vi "Main.vi"() -> ()   [LabVIEW 2014]
uses:
  <vilib>/Instr/_visa.llb/VISA Configure Serial Port (Instr).vi
panel:
  in  "Sim Delay":u32(slide)=100 scale=0.0..2000.0
  in  "조작모드":string(combo)="기본"
  out "Serial Loop":i32=157
  in  "Serial Settings":T1={"baud rate"=9600, "data bits"=8, "parity"=enum."None", "stop bits"=10, "flow control"=0} {"flow control" items=["None"=0, "XON/XOFF"=1, "RTS/CTS"=2, "DTR/DSR"=4]; "stop bits" items=["1.0"=10, "1.5"=15, "2.0"=20]; "data bits" min=5 max=8 step=1; "baud rate" items=["75"=75, "110"=110, "134"=134, "150"=150, "300"=300, "600"=600, "1200"=1200, "1800"=1800, "2400"=2400, "4800"=4800, "7200"=7200, "9600"=9600, "14400"=14400, "19200"=19200, "28800"=28800, "38400"=38400, "56000"=56000, "57600"=57600, "115200"=115200, "128000"=128000, "230400"=230400]}
  in  "VISA 2":refnum<visa-resource-name>="COM4"
  in  "VISA 1":refnum<visa-resource-name>="COM3"
  out "Running 2":bool=TRUE caption="Running"
  in  "재생 버튼":bool
  out "Running":bool=TRUE
  in  "Serial Delay":u32(slide)=1000 scale=0.0..2000.0
  out "C축":dbl(knob)=10.0 scale=0.0..10.0
  out "R축":dbl(knob) scale=0.0..10.0
  out "L축":dbl(knob) scale=0.0..10.0
  out "Wrtie":string
  out "Axis":string
  out "위치 좌표 값 그래프":dbl[][](graph)=[[127.0, 127.0, 127.0], [127.0, 127.0, 127.0], [127.0, 127.0, 127.0], [127.0, 127.0, 127.0], [127.0, 127.0, 127.0], [127.0, 127.0, 127.0], [127.0, 127.0, 127.0], [127.0, 127.0, 127.0], [127.0, 127.0, 127.0], [127.0, 127.0, 127.0], [127.0, 127.0, 127.0], [127.0, 127.0, 127.0], [127.0, 127.0, 127.0], [127.0, 127.0, 127.0], [127.0, 127.0, 127.0], [127.0, 127.0, 127.0], [127.0, 127.0, 127.0], [127.0, 127.0, 127.0], [127.0, 127.0, 127.0], [127.0, 127.0, 127.0], [127.0, 127.0, 127.0], [127.0, 127.0, 127.0], [127.0, 127.0, 127.0], [127.0, 127.0, 127.0], [127.0, 127.0, 127.0], [127.0, 127.0, 127.0], [127.0, 127.0, 127.0], [127.0, 127.0, 127.0], [127.0, 127.0, 127.0], [127.0, 127.0, 127.0], [127.0, 127.0, 127.0], [127.0, 127.0, 127.0], [127.0, 127.0, 127.0], [127.0, 127.0, 127.0], [127.0, 127.0, 127.0], [127.0, 127.0, 127.0], [127.0, 127.0, 127.0], [127.0, 127.0, 127.0], [127.0, 127.0, 127.0], [127.0, 127.0, 127.0], [127.0, 127.0, 127.0], [127.0, 127.0, 127.0], [127.0, 127.0, 127.0], [127.0, 127.0, 127.0], [127.0, 127.0, 127.0], [127.0, 127.0, 127.0], [127.0, 127.0, 127.0], [127.0, 127.0, 127.0], [127.0, 127.0, 127.0], [127.0, 127.0, 127.0], [127.0, 127.0, 127.0], [127.0, 127.0, 127.0], [127.0, 127.0, 127.0], [127.0, 127.0, 127.0], [127.0, 127.0, 127.0], [127.0, 127.0, 127.0], [127.0, 127.0, 127.0], [127.0, 127.0, 127.0], [127.0, 127.0, 127.0], [127.0, 127.0, 127.0], [127.0, 127.0, 127.0], [127.0, 127.0, 127.0], [127.0, 127.0, 127.0], [127.0, 127.0, 127.0], [127.0, 127.0, 127.0], [127.0, 127.0, 127.0], [127.0, 127.0, 127.0], [127.0, 127.0, 127.0], [127.0, 127.0, 127.0], [127.0, 127.0, 127.0], [127.0, 127.0, 127.0], [127.0, 127.0, 127.0], [127.0, 127.0, 127.0], [127.0, 127.0, 127.0], [127.0, 127.0, 127.0], [127.0, 127.0, 127.0], [127.0, 127.0, 127.0], [127.0, 127.0, 127.0], [127.0, 127.0, 127.0], [127.0, 127.0, 127.0], [127.0, 127.0, 127.0], [127.0, 127.0, 127.0], [127.0, 127.0, 127.0], [127.0, 127.0, 127.0], [127.0, 127.0, 127.0], [127.0, 127.0, 127.0], [127.0, 127.0, 127.0], [127.0, 127.0, 127.0], [127.0, 127.0, 127.0], [127.0, 127.0, 127.0], [127.0, 127.0, 127.0], [127.0, 127.0, 127.0], [127.0, 127.0, 127.0], [127.0, 127.0, 127.0], [127.0, 127.0, 127.0], [127.0, 127.0, 127.0], [127.0, 127.0, 127.0], [127.0, 127.0, 127.0], [127.0, 127.0, 127.0], [127.0, 127.0, 127.0], [127.0, 127.0, 127.0], [127.0, 127.0, 127.0], [127.0, 127.0, 127.0], [127.0, 127.0, 127.0], [127.0, 127.0, 127.0], [127.0, 127.0, 127.0], [127.0, 127.0, 127.0], [127.0, 127.0, 127.0], [127.0, 127.0, 127.0], [127.0, 127.0, 127.0], [127.0, 127.0, 127.0], [127.0, 127.0, 127.0], [127.0, 127.0, 127.0], [127.0, 127.0, 127.0], [127.0, 127.0, 127.0], [127.0, 127.0, 127.0], [127.0, 127.0, 127.0], [127.0, 127.0, 127.0], [127.0, 127.0, 127.0], [127.0, 127.0, 127.0], [127.0, 127.0, 127.0], [127.0, 127.0, 127.0], [127.0, 127.0, 127.0], [127.0, 127.0, 127.0], [127.0, 127.0, 127.0], [127.0, 127.0, 127.0], [127.0, 127.0, 127.0], [127.0, 127.0, 127.0], [127.0, 127.0, 127.0], [127.0, 127.0, 127.0], [127.0, 127.0, 127.0], [127.0, 127.0, 127.0], [127.0, 127.0, 127.0], [127.0, 127.0, 127.0], [127.0, 127.0, 127.0], [127.0, 127.0, 127.0], [127.0, 127.0, 127.0], [127.0, 127.0, 127.0], [127.0, 127.0, 127.0], [127.0, 127.0, 127.0], [127.0, 127.0, 127.0], [127.0, 127.0, 127.0], [127.0, 127.0, 127.0], [127.0, 127.0, 127.0], [127.0, 127.0, 127.0], [127.0, 127.0, 127.0], [127.0, 127.0, 127.0], [127.0, 127.0, 127.0], [127.0, 127.0, 127.0], [127.0, 127.0, 127.0], [127.0, 127.0, 127.0], [127.0, 127.0, 127.0], [127.0, 127.0, 127.0], [127.0, 127.0, 127.0], [127.0, 127.0, 127.0], [127.0, 127.0, 127.0], [127.0, 127.0, 127.0], [127.0, 127.0, 127.0]]
  in  "Error In":errorcluster
  in  "포트":u16=50
  in  "IP":string="127.0.0.1"
  in  "Running Game":string="DiRT 3"
  out "Sim Loop":i32=157
  in  "Simtools ON":bool
  in  "STOP":bool
  out "Error Out":errorcluster={"status"=TRUE, "code"=-1074360311, "source"="IMAQdx Open Camera.vi"}
  # "지도교수 : 손종원 교수님, 윤한재 교수님, 노일수 교수님  개발자 : 하기봉, 박재우"
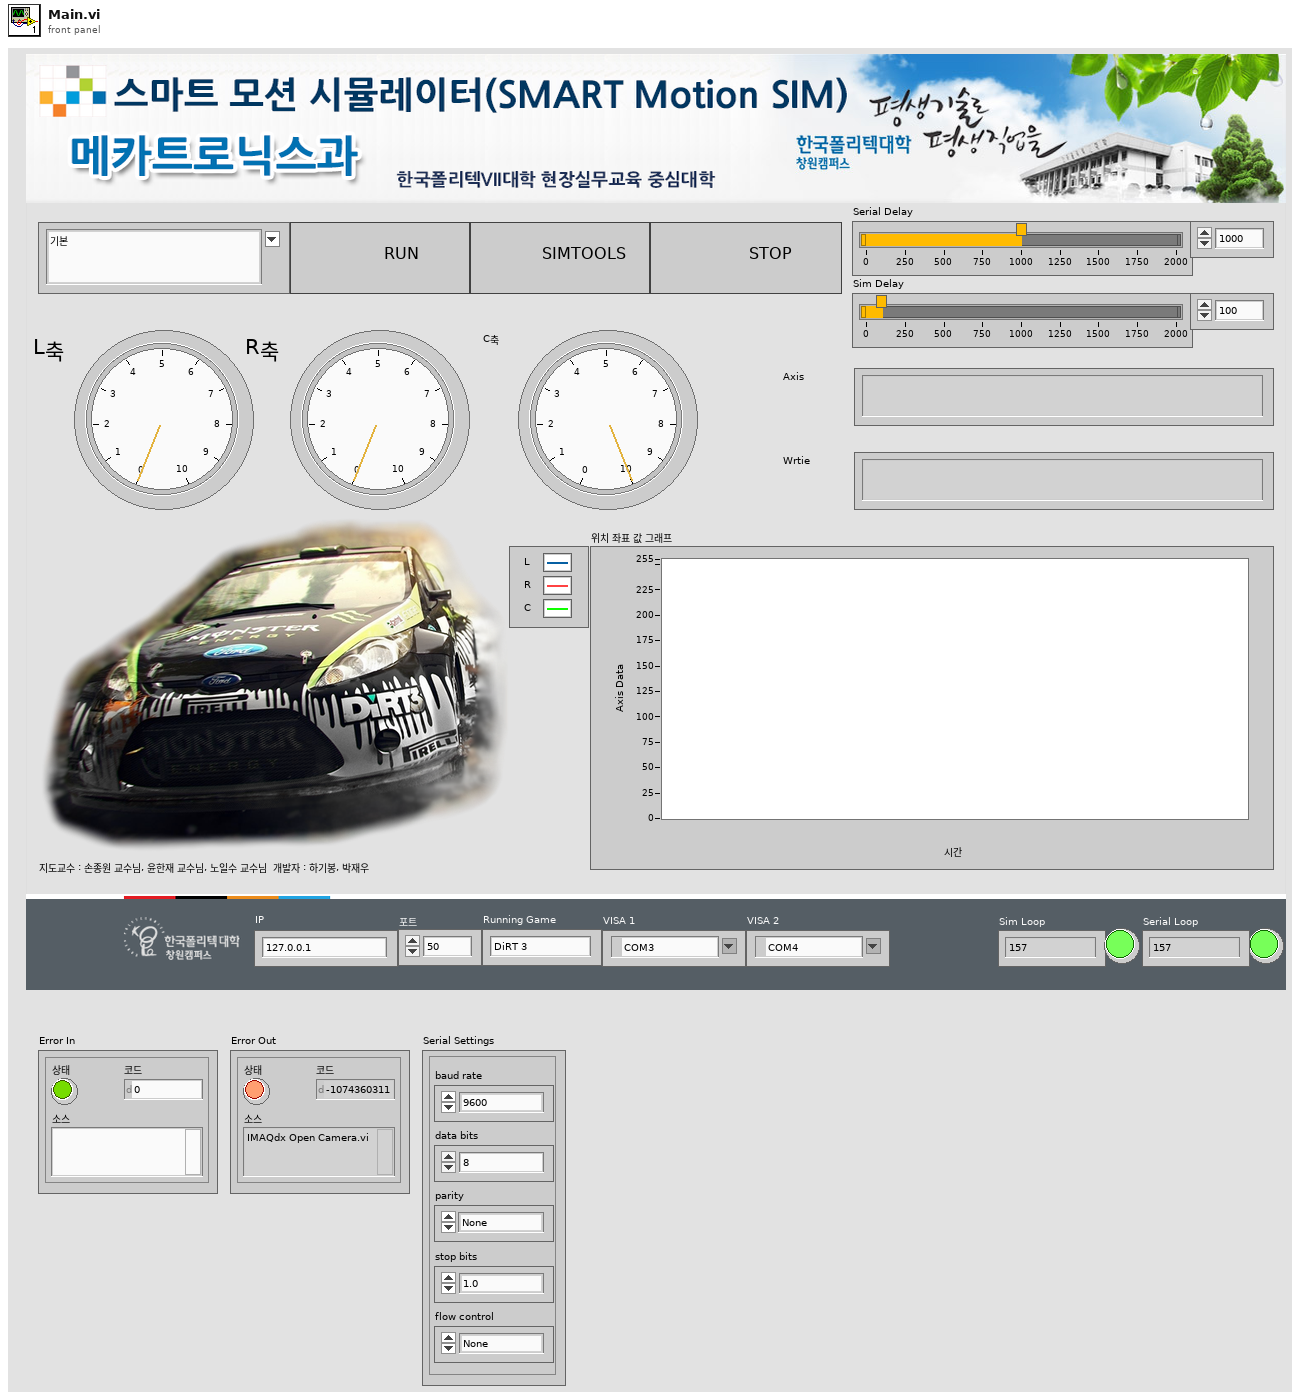
[diagram p1: front panel]
types:
  T1 = cluster{"baud rate":u32, "data bits":u16, "parity":enum16{"None", "Odd", "Even", "Mark", "Space"}, "stop bits":u16, "flow control":u16}
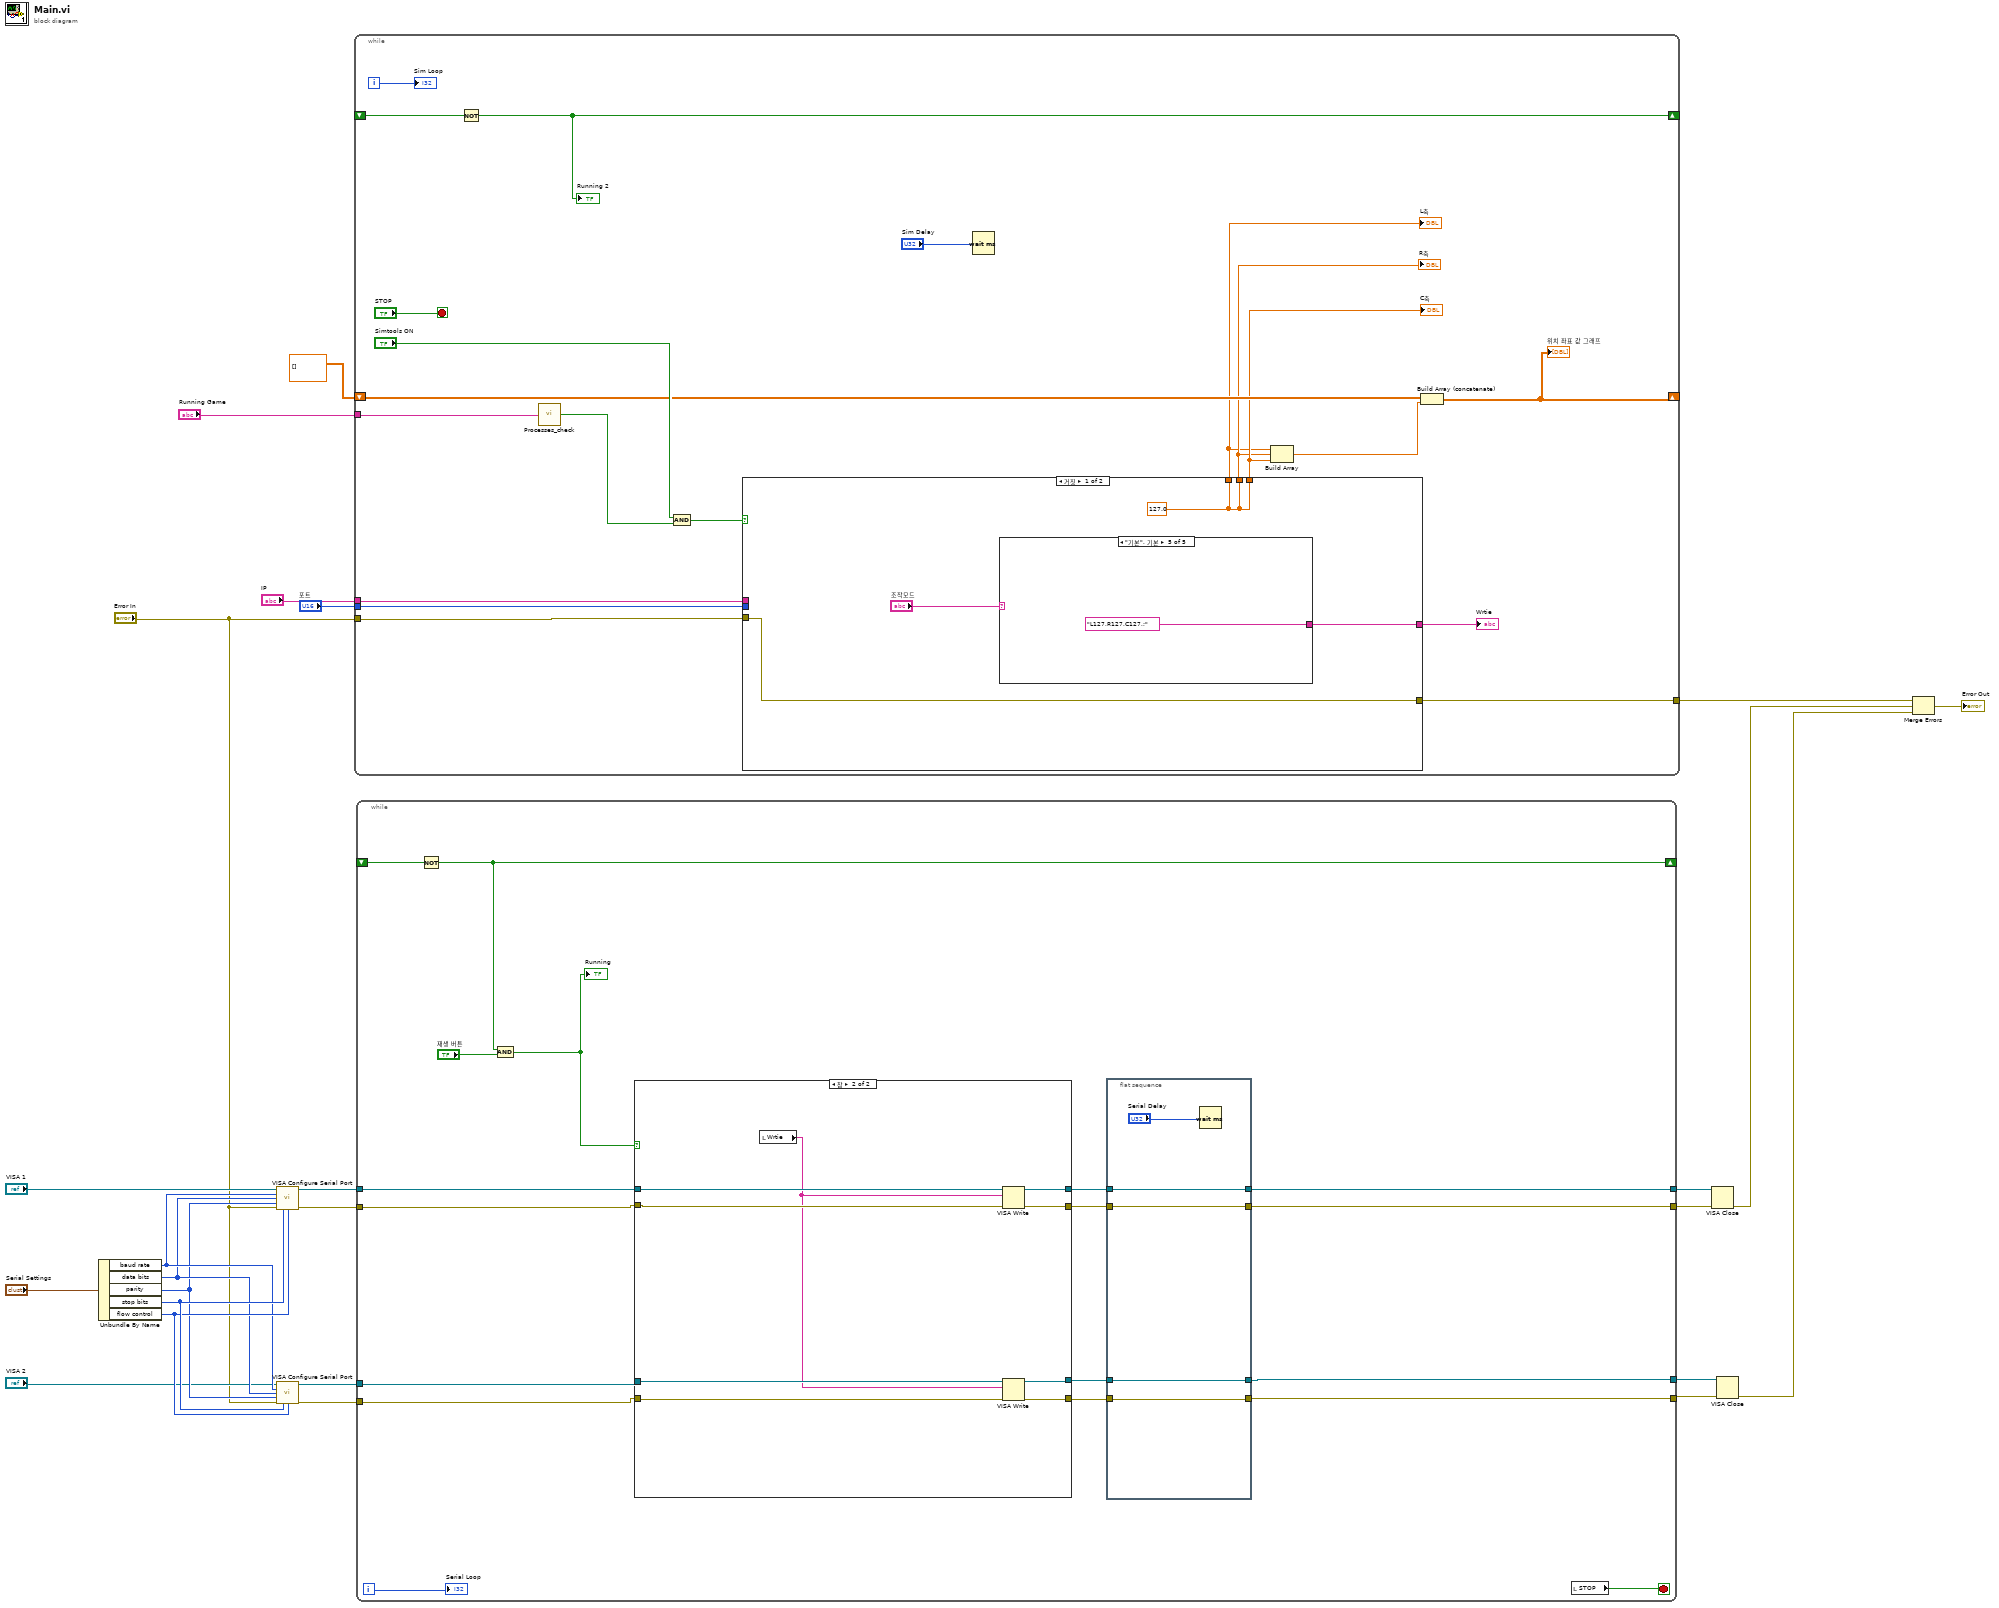
[diagram p0: block diagram]
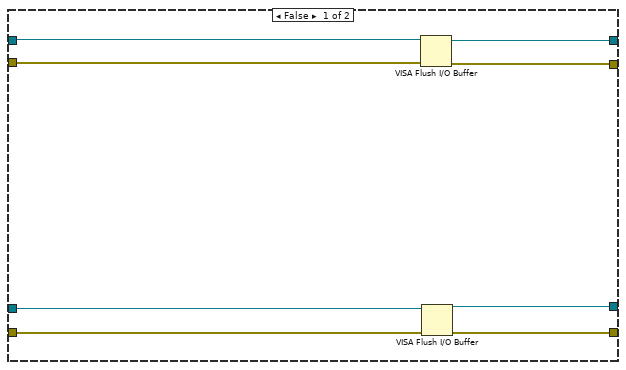
[diagram p2: hidden frame]
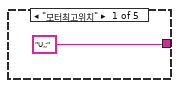
[diagram p3: hidden frame]
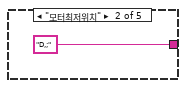
[diagram p4: hidden frame]
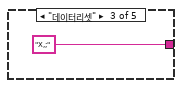
[diagram p5: hidden frame]
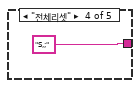
[diagram p6: hidden frame]
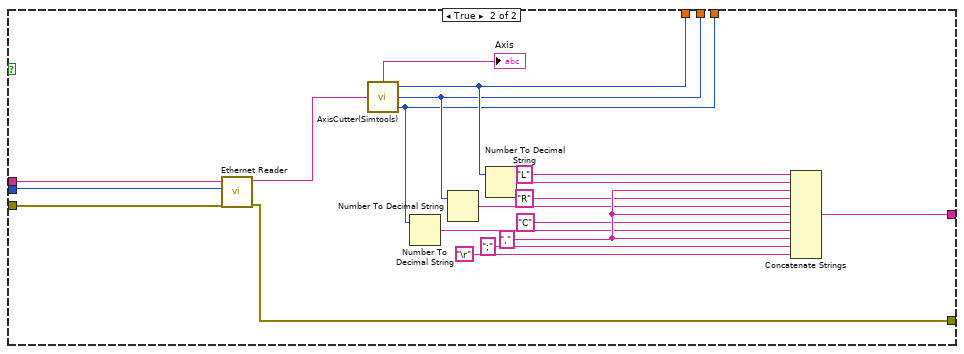
[diagram p7: hidden frame]
diagram:
  n1 = Unbundle By Name("Serial Settings") -> ("baud rate"=w16:u32, "data bits"=w15:u16, "parity"=w14:enum16{"None", "Odd", "Even", "Mark", "Space"}, "stop bits"=w18:u16, "flow control"=w17:u16)
  n2 = call-poly "VISA Configure Serial Port"("VISA resource name"="VISA 1", "baud rate (9600)"=w16, "data bits (8)"=w15, "parity (0:none)"=w14, "error in (no error)"="Error In", "stop bits (10: 1 bit)"=w18, "flow control (0:none)"=w17) -> ("VISA resource name out"=w11:refnum<visa-resource-name>, "error out"=w8:errorcluster)  [unwired: 7 in]
  n3 = call-poly "VISA Configure Serial Port"("VISA resource name"="VISA 2", "baud rate (9600)"=w16, "data bits (8)"=w15, "parity (0:none)"=w14, "error in (no error)"="Error In", "stop bits (10: 1 bit)"=w18, "flow control (0:none)"=w17) -> ("VISA resource name out"=w10:refnum<visa-resource-name>, "error out"=w9:errorcluster)  [unwired: 7 in]
  n4 = while {
    tunnel: "Running Game" -> [w37]
    tunnel: "포트" -> [w41]
    tunnel: "IP" -> [w40]
    tunnel: "Error In" -> [w39]
    tunnel: [w38] -> w21
    shift-right: [w33] -> _
    shift-left: dbl[][] [] -> [w35]
    shift-right: [w27] -> _
    shift-left: _ -> [w28]
    i -> [w44]
    stop <- "STOP" stop-if-true
    n5 = Not(x=w28) -> (.not. x?=w27:bool)
    "Running 2" <- w27
    n6 = call "Processes_check.vi"("검색 내용"=w37) -> ("불리언"=w36:bool)
    n7 = And(x="Simtools ON", y=w36) -> (x .and. y?=w42:bool)
    n8 = case shown="거짓" w42 {
      tunnel: w41 -> [_ w71]
      tunnel: w40 -> [_ w72]
      tunnel: w39 -> [w49 w70]
      tunnel: [w49 w69] -> w38
      tunnel: [w48 w58] -> w29
      tunnel: [w48 w57] -> w30
      tunnel: [w48 w56] -> w31
      tunnel: [w47 w55] -> w32
      frame False {
        w48 = 127.0
        n9 = case shown="\"기본\", 기본" "조작모드" {
          tunnel: ["U,;" "D,;" "X,;" "S,;" "L127,R127,C127,;"] -> w47
          frame "모터최고위치" {
          }
          frame "모터최저위치" {
          }
          frame "데이터리셋" {
          }
          frame "전체리셋" {
          }
          frame "기본", Default {
          }
        }
      }
      frame True {
        w65 = ","
        n10 = call "Ethernet Reader.vi"("IP"=w72, "포트"=w71, "에러 입력(에러 없음)"=w70) -> ("Axis"=w73:string, "에러 출력"=w69:errorcluster)  [unwired: 5 in]
        n11 = call "AxisCutter(Simtools).vi"("수신"=w73) -> ("Axis"=→"Axis":string, "L"=w58:i32, "R"=w57:i32, "C"=w56:i32)
        n12 = Number To Decimal String(number=w56) -> (decimal integer string=w61:string)  [unwired: 1 in]
        n13 = Number To Decimal String(number=w57) -> (decimal integer string=w63:string)  [unwired: 1 in]
        n14 = Number To Decimal String(number=w58) -> (decimal integer string=w66:string)  [unwired: 1 in]
        n15 = Concatenate Strings("L", w66, w65, "R", w63, w65, "C", w61, w65, ";", "\r") -> (w55:string)
      }
    }
    "Wrtie" <- w32
    "L축" <- w29
    "R축" <- w30
    "C축" <- w31
    n16 = Wait (ms)(milliseconds to wait="Sim Delay") -> ()  [unwired: 1 out]
    n17 = Build Array(w29, w30, w31) -> (w34:dbl[])
    n18 = Build Array (concatenate)(w35, w34) -> (w33:dbl[][])
    "위치 좌표 값 그래프" <- w33
    "Sim Loop" <- w44
  }
  n19 = while {
    shift-right: [w85] -> _
    shift-left: _ -> [w86]
    tunnel: w11 -> [w83]
    tunnel: w10 -> [w82]
    tunnel: w9 -> [w81]
    tunnel: w8 -> [w80]
    tunnel: [w79] -> w6
    tunnel: [w78] -> w5
    tunnel: [w77] -> w4
    tunnel: [w76] -> w3
    i -> [w75]
    stop <- w74 stop-if-true
    n20 = Not(x=w86) -> (.not. x?=w85:bool)
    n21 = And(x=w85, y="재생 버튼") -> (x .and. y?=w84:bool)
    "Running" <- w84
    n22 = case shown="참" w84 {
      tunnel: [w104 w113] -> w91
      tunnel: [w103 w112] -> w90
      tunnel: w83 -> [w102 w111]
      tunnel: w82 -> [w100 w110]
      tunnel: w81 -> [w99 w109]
      tunnel: w80 -> [w101 w108]
      tunnel: [w97 w107] -> w89
      tunnel: [w98 w106] -> w88
      frame False {
        n23 = VISA Flush I/O Buffer(VISA resource name=w102, error in (no error)=w101) -> (VISA resource name out=w104:refnum<visa-resource-name>, error out=w103:errorcluster)  [unwired: 1 in]
        n24 = VISA Flush I/O Buffer(VISA resource name=w100, error in (no error)=w99) -> (VISA resource name out=w97:refnum<visa-resource-name>, error out=w98:errorcluster)  [unwired: 1 in]
      }
      frame True {
        n25 = local read "Wrtie"() -> (w105:string)
        n26 = VISA Write(VISA resource name=w111, write buffer=w105, error in (no error)=w108) -> (VISA resource name out=w113:refnum<visa-resource-name>, error out=w112:errorcluster)  [unwired: 1 out]
        n27 = VISA Write(VISA resource name=w110, write buffer=w105, error in (no error)=w109) -> (VISA resource name out=w107:refnum<visa-resource-name>, error out=w106:errorcluster)  [unwired: 1 out]
      }
    }
    n28 = flat-sequence {
      tunnel: w91 -> [w96]
      tunnel: w90 -> [w94]
      tunnel: [w96] -> w76
      tunnel: w89 -> [w93]
      tunnel: w88 -> [w92]
      tunnel: [w94] -> w79
      tunnel: [w93] -> w77
      tunnel: [w92] -> w78
      frame #0 {
        n29 = Wait (ms)(milliseconds to wait="Serial Delay") -> ()  [unwired: 1 out]
      }
    }
    n30 = local read "STOP"() -> (w74:bool)
    "Serial Loop" <- w75
  }
  n31 = VISA Close(VISA resource name=w3, error in (no error)=w6) -> (error out=w2:errorcluster)
  n32 = VISA Close(VISA resource name=w4, error in (no error)=w5) -> (error out=w1:errorcluster)
  n33 = Merge Errors(w21, w2, w1) -> (→"Error Out":errorcluster)
